vi "LVFunction_Imop_Get Sequence.vi"(0 "tab Haso Data":refnum<class "HasoData.lvclass">[](array[class]), 5 "path":path, 11 "error in (no error)":errorcluster) -> (4 "tab HASO DATA":refnum<class "HasoData.lvclass">[](array[class]), 15 "error out":errorcluster)   [LabVIEW 2020]
doc: "Load a HasoData array from file.\n\n--------------------------------------------------------------------------------\n\n<B>HasoDataIn</B> : Array of HasoData object.\n\n<B>HasoDataOut</B> : Array of HasoData object.\n\n<B>sequence_file_path</B> : Absolute path to sequence file.\n\n<B>ErrorIn</B> : Error\n\n<B>ErrorOut</B> : Error"
uses:
  HasoData.lvclass
  LVClass_HasoData Read HasoData - property.vi
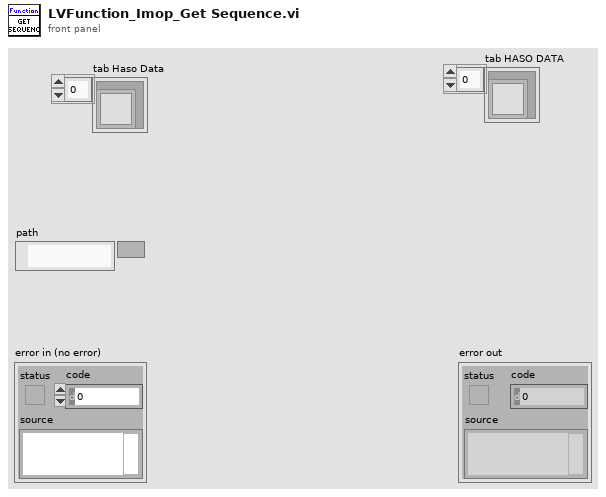
[diagram p1: front panel]
types:
  T1 = typedef "ClassID.ctl" = i64
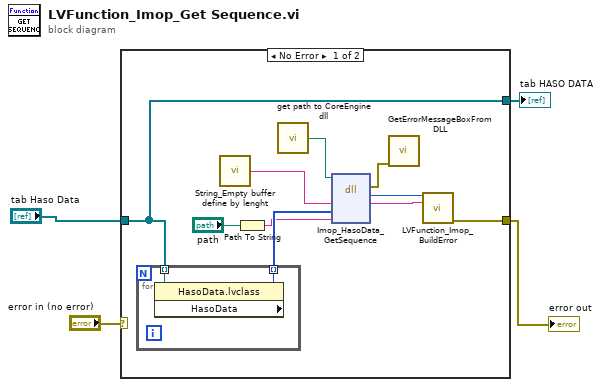
[diagram p0: block diagram]
diagram:
  n1 = case shown="No Error" "error in (no error)" {
    selector: "error in (no error)" -> [_ w18]
    tunnel: [w12 w18] -> w3
    tunnel: "tab Haso Data" -> [w5 w17]
    tunnel: [w5 w17] -> w1
    frame No Error {
      n2 = for {
        tunnel: w5 -> [w16] mode=indexing
        tunnel: [w15] -> w8 mode=indexing
        n3 = property class="HasoData.lvclass"(reference=w16) -> ("HasoData"=w15:T1)  [unwired: 1 in, 2 out]
      }
      n4 = call "String_Empty buffer define by lenght.vi"() -> ("Empty buffer"=w9:string)  [unwired: 1 in]
      n5 = Path To String(path="path") -> (string=w7:string)
      n6 = call "get path to CoreEngine dll.vi"() -> ("path to wavekit library"=w11:path)  [unwired: 14 in, 1 out]
      n7 = dll-call lib="D:/2_trunk/Soft_haso/ImOpCoreEngine4_LV2011/DLLs/ImopEngine4_vc100.dll" fn="Imop_HasoData_GetSequence"(path in=w11, "message"=w9, "HasoData"=w8, "SequenceFilePath"=w7) -> (error out=w10:errorcluster, "return type"=w14:i32, "message"=w13:string)  [unwired: 4 in, 1 out]
      n8 = call "GetErrorMessageBoxFromDLL.vi"("error IN"=w10) -> ()  [unwired: 10 in, 1 out]
      n9 = call "LVFunction_Imop_BuildError.vi"("code"=w14, "String to Prepend to source (\"\")"=w13) -> ("error out"=w12:errorcluster)  [unwired: 13 in]
    }
    frame Error {
    }
  }
  "error out" <- w3
  "tab HASO DATA" <- w1
